vi "Cleanup.vi"(8 "error in (no error)":errorcluster, 11 "ByRef Base in":refnum<class "ByRef Base.lvclass">) -> (0 "error out":errorcluster)   [LabVIEW 2012, in "ByRef Base.lvclass"]
uses:
  ByRef Base.lvclass
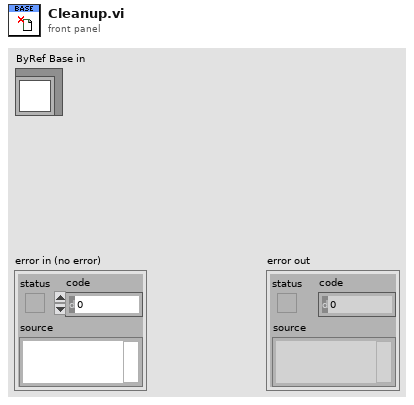
[diagram p1: front panel]
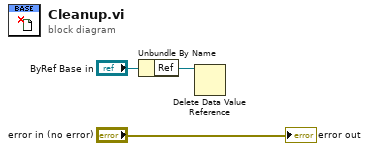
[diagram p0: block diagram]
diagram:
  n1 = Unbundle By Name("ByRef Base in") -> ("Ref"=w1:refnum<data-value>)
  n2 = Delete Data Value Reference(data value reference=w1) -> ()  [unwired: 1 in, 2 out]
  "error out" <- "error in (no error)"
